vi "Configure Auto Focusing.vi"(0 "VISA Resource Name":refnum<visa-resource-name>, 5 "Device Number (1)":i32=1, 7 "Autofocus (0: Real-time)":enum16{"Real-Time", "One-Shot", "Off"}(ring), 11 "error in (no error)":errorcluster {"code" format="%.0x"}) -> (4 "VISA Resource Name Out":refnum<visa-resource-name>, 15 "error out":errorcluster {"code" format="%.0x"})   [LabVIEW 2018, in "Olympus IX BX Series.lvlib"]
doc: "Starts / stops autofocusing.\n\nNotes:\n(1) The movement VIs can not move the stage while autofocusing is controlled with this VI. (Return a busy status).\n\n(2) Stops autofocusing always suspends autofocusing.\n\n(3) Autofocusing is not performed properly unless the stage near/far limit and the AF near/far limit are set properly.\n\n(4) Autofocusing is not performed properly unless the AF parameter is specified properly with the Select AF parameter table VI."
uses:
  Olympus IX BX Series.lvlib
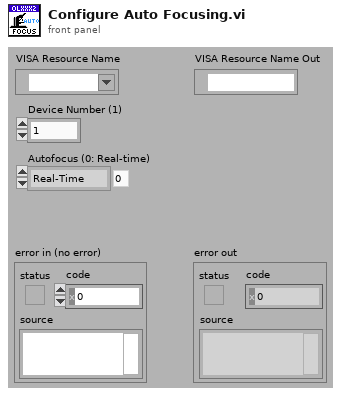
[diagram p1: front panel]
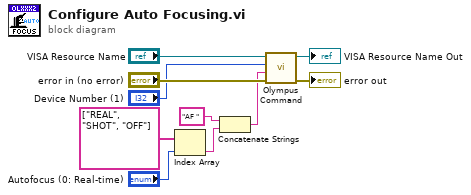
[diagram p0: block diagram]
diagram:
  n1 = Index Array(array=string[] ["REAL", "SHOT", "OFF"], index="Autofocus (0: Real-time)") -> (element=w5:string)
  n2 = Concatenate Strings("AF " ("format string"), w5) -> (w3:string)
  n3 = call "Olympus Command.vi"("error in (no error)"="error in (no error)", "Command string"=w3, "Device Number (1)"="Device Number (1)", "VISA Resource Name"="VISA Resource Name") -> ("error out"=→"error out":errorcluster, "VISA Resource Name Out"=→"VISA Resource Name Out":refnum<visa-resource-name>)  [unwired: 5 in, 1 out]
